vi "generateTempFile.vi"(8 "error in (no error)":errorcluster, 11 "MS-Word in":refnum<class "MS-Word.lvclass">) -> (0 "error out":errorcluster, 2 "Temporary File Path":path, 3 "MS-Word out":refnum<class "MS-Word.lvclass">)   [LabVIEW 2017, in "LabVIEW NPOI.lvlib" / "MS-Word.lvclass"]
uses:
  MS-Word.lvclass
  C:/Users/Neo/Desktop/Dev_Tools_BR/LabVIEW_NPOI/src/LabVIEW NPOI/Document/Document.lvclass
  Document/Document.lvclass
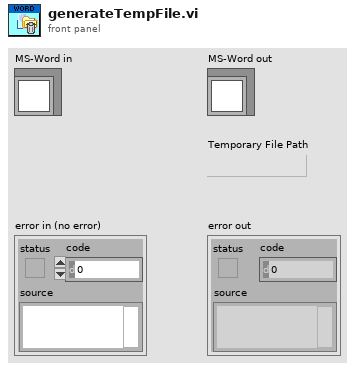
[diagram p1: front panel]
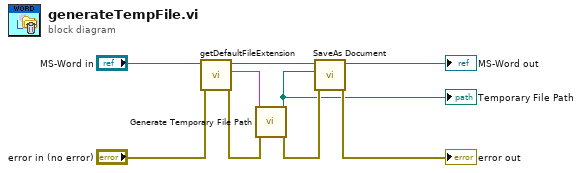
[diagram p0: block diagram]
diagram:
  n1 = call-dynamic "getDefaultFileExtension.vi"("error in (no error)"="error in (no error)", "MS-Word in"="MS-Word in") -> ("error out"=w4:errorcluster, "Default File Extension"=w9:string, "MS-Word out"=w8:refnum<class "MS-Word.lvclass">)  [unwired: 7 in]
  n2 = call <vilib>:"Generate Temporary File Path.vi"("error in (no error)"=w4, "Temporary File Extension (tmp)"=w9) -> ("error out"=w3:errorcluster, "Unique Temporary File Path"=w1:path)  [unwired: 8 in]
  "Temporary File Path" <- w1
  n3 = call "SaveAs Document.vi"("error in (no error)"=w3, "File Path"=w1, "Document in"=w8) -> ("error out"=→"error out":errorcluster, "Document out"=→"MS-Word out":refnum<class "MS-Word.lvclass">)  [unwired: 7 in]
